vi "AssertAlmostEqual_Tests.vi"(11 "error in (no error)":errorcluster) -> (15 "error out":errorcluster)   [LabVIEW 2016, in "DronaTest.lvlib"]
uses:
  DronaTest.lvlib
  APIs/Stimulus/VI/MakeVIFrontMost.vi
  APIs/Assert/AssertControlValue/AlmostEqual.vi
  <vilib>/addons/_JKI Toolkits/Caraya/classes/Assert/Assert Error.vi
  <vilib>/addons/_JKI Toolkits/Caraya/classes/Test/Test.lvclass
  Drona.lvlib
  APIs/Assert/AssertControlValue/AssertControlValue.lvlib
  <vilib>/addons/_JKI Toolkits/Caraya/classes/Assert/Assert.lvclass
  APIs/Stimulus/VI/VI.lvlib
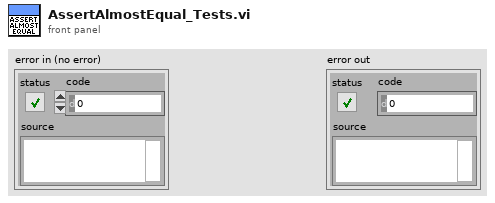
[diagram p1: front panel]
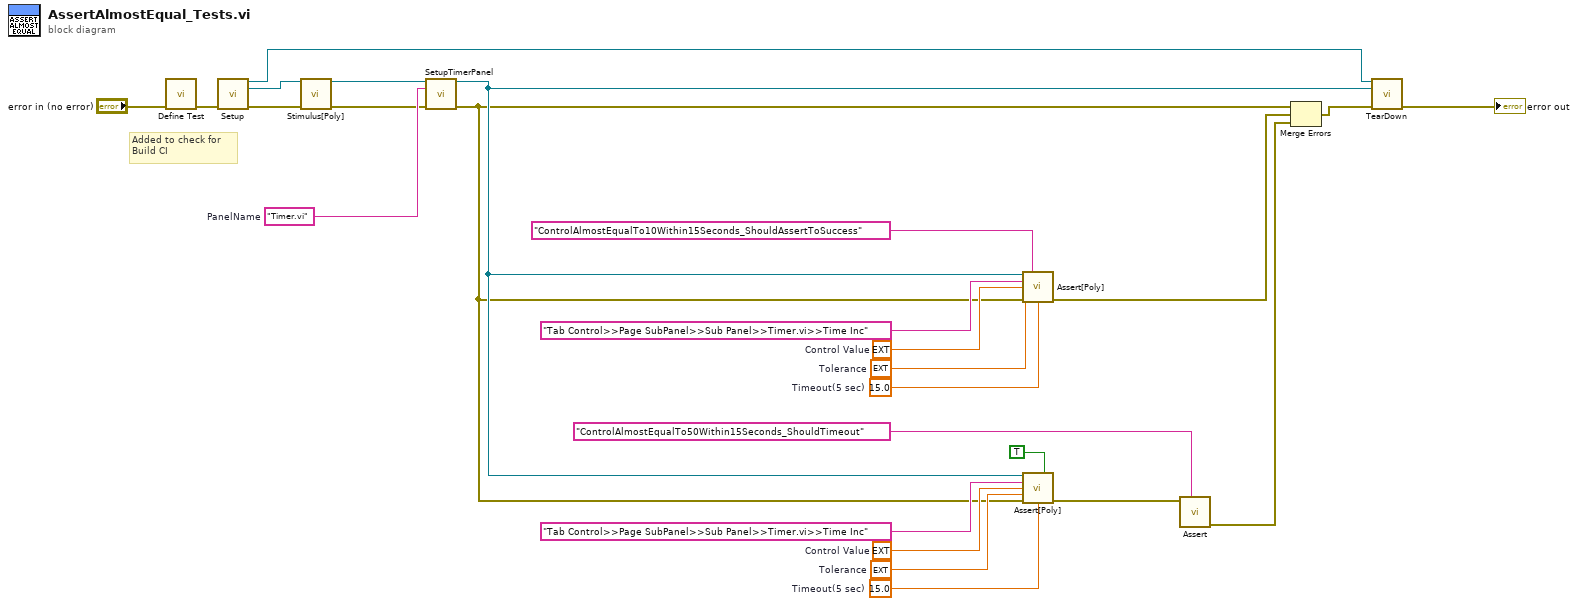
[diagram p0: block diagram]
diagram:
  w11 = "Timer.vi"  # PanelName
  w16 = ext 0.5  # Tolerance
  w17 = ext 0.5  # Tolerance
  w21 = 15.0  # Timeout(5 sec)
  w20 = ext 50.0  # Control Value
  w22 = 15.0  # Timeout(5 sec)
  w23 = ext 10.0  # Control Value
  # "Added to check for \nBuild CI"
  n1 = call <vilib>:"Define Test.vi"("error in (no error)"="error in (no error)") -> ("error out"=w15:errorcluster)  [unwired: 10 in]
  n2 = call "Setup.vi"("error in (no error)"=w15) -> ("Application Ref"=w12:refnum<vi>, "VI out"=w3:refnum<vi>, "error out"=w4:errorcluster)  [unwired: 12 in]
  n3 = call-poly "Stimulus[Poly].vi"("VI Reference In"=w3, "error in"=w4) -> ("VI Reference Out"=w2:refnum<vi>, "error out"=w1:errorcluster)  [unwired: 12 in]
  n4 = call "SetupTimerPanel.vi"("VI in"=w2, "Panel Name"=w11, "error in (no error)"=w1) -> ("VI out"=w10:refnum<vi>, "error out"=w9:errorcluster)  [unwired: 11 in]
  n5 = call-poly "Assert[Poly].vi"("VI Reference In"=w10, "Test Label"="ControlAlmostEqualTo10Within15Seconds_ShouldAssertToSuccess" ("string"), "Control Path"="Tab Control>>Page SubPanel>>Sub Panel>>Timer.vi>>Time Inc", "Control Value"=w23, "Tolerance"=w17, "Error In"=w9, "Timeout(5 sec)"=w22) -> ("Error Out"=w24:errorcluster)  [unwired: 7 in, 1 out]
  n6 = call-poly "Assert[Poly].vi"("VI Reference In"=w10, "Assert Only? (F)"=TRUE, "Control Path"="Tab Control>>Page SubPanel>>Sub Panel>>Timer.vi>>Time Inc", "Control Value"=w20, "Tolerance"=w16, "Error In"=w9, "Timeout(5 sec)"=w21) -> ("Error Out"=w5:errorcluster)  [unwired: 7 in, 1 out]
  n7 = call-poly <vilib>:"Assert.vi"("Label"="ControlAlmostEqualTo50Within15Seconds_ShouldTimeout" ("string"), "Error?"=w5) -> ("error out"=w7:errorcluster)  [unwired: 9 in]
  n8 = Merge Errors(w9, w24, w7) -> (w14:errorcluster)
  n9 = call "TearDown.vi"("Application Ref"=w12, "VI in"=w10, "error in (no error)"=w14) -> ("error out"=→"error out":errorcluster)  [unwired: 12 in]
